vi "Set External Trigger Termination.vi"(11 "uiTermination":u32) -> (3 "function return":u32)   [LabVIEW 2018, in "Copy of Andor SDK.lvlib"]
doc: "EXPNETTYPE unsigned int WINAPI SetExternalTriggerTermination(at_u32 uiTermination);"
uses:
  Copy of Andor SDK.lvlib
  <userlib>/Andor SDK/ATMCD32D.dll
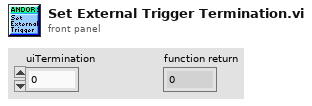
[diagram p1: front panel]
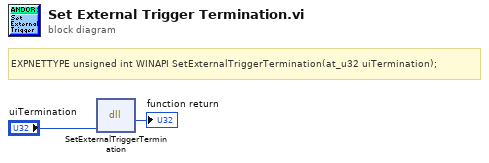
[diagram p0: block diagram]
diagram:
  # "EXPNETTYPE unsigned int WINAPI SetExternalTriggerTermination(at_u32 uiTermination);"
  n1 = dll-call lib="C:/Program Files (x86)/National Instruments/LabVIEW 2018/user.lib/Andor SDK/ATMCD32D.*" fn="SetExternalTriggerTermination"("uiTermination"="uiTermination") -> (→"function return":u32)  [unwired: 4 in, 2 out]
